vi "Dictionary Test - 001.vi"(8 "error in (no error)":errorcluster) -> (0 "error out":errorcluster, 2 "pass":bool)   [LabVIEW 2009]
uses:
  source/library/Dictionary Update/Dictionary Update (by value).vi
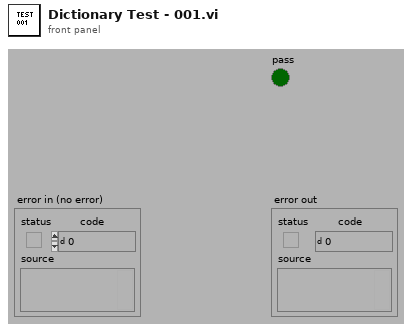
[diagram p1: front panel]
types:
  T1 = typedef "Dictionary Object RefNum.ctl" = refnum<k1>
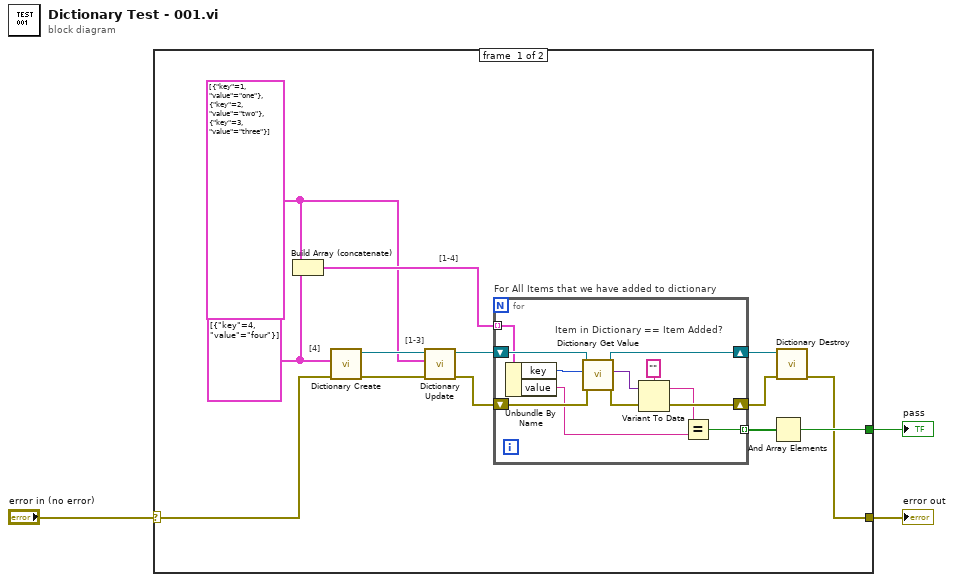
[diagram p0: block diagram]
diagram:
  n1 = case shown="No Error" "error in (no error)" {
    selector: "error in (no error)" -> [w9 w29]
    tunnel: [w7 w29] -> w1
    tunnel: [w8 _] -> w3
    frame #0 {
      w5 = cluster{"key":i32, "value":string}[] [{"key"=4, "value"="four"}] ("initial dictionary (empty)")
      w4 = cluster{"key":i32, "value":string}[] [{"key"=1, "value"="one"}, {"key"=2, "value"="two"}, {"key"=3, "value"="three"}] ("dictionary with updates")
      # "[1-4]"
      # "[4]"
      # "[1-3]"
      n2 = Build Array (concatenate)(w4, w5) -> (w6:cluster{"key":i32, "value":string}[])
      n3 = call "Dictionary Create.vi"("error in (no error)"=w9, "initial dictionary (empty)"=w5) -> ("error out"=w15:errorcluster, "dictionary out"=w16:T1)  [unwired: 8 in]
      n4 = call-poly "Dictionary Update.vi"("error in (no error)"=w15, "dictionary with updates"=w4, "dictionary"=w16) -> ("error out"=w13:errorcluster, "dictionary out"=w14:T1)  [unwired: 6 in, 1 out]
      n5 = for "For All Items that we have added to dictionary" {
        tunnel: w6 -> [w18] mode=indexing
        shift-right: [w25] -> w12
        shift-left: w14 -> [w26]
        shift-right: [w22] -> w11
        shift-left: w13 -> [w27]
        tunnel: [w17] -> w10 mode=indexing
        # "Item in Dictionary == Item Added?"
        n6 = Unbundle By Name(w18) -> ("key"=w28:i32, "value"=w19:string)
        n7 = call "Dictionary Get Value.vi"("error in"=w27, "key"=w28, "dictionary"=w26) -> ("error out"=w23:errorcluster, "value"=w24:variant, "dictionary out"=w25:T1)  [unwired: 5 in, 1 out]
        n8 = Variant To Data(error in=w23, Variant=w24, type="" ("value")) -> (error out=w22:errorcluster, data=w20:string)
        n9 = Equal?(x=w20, y=w19) -> (x = y?=w17:bool)
      }
      n10 = And Array Elements(Boolean array=w10) -> (logical AND=w8:bool)
      n11 = call "Dictionary Destroy.vi"("error in (no error)"=w11, "dictionary"=w12) -> ("error out"=w7:errorcluster)  [unwired: 9 in]
    }
    frame #1 {
    }
  }
  "pass" <- w3
  "error out" <- w1
